vi "Update DUT Status.vi"(6 "Position":i32, 7 "Ignore State (true)":bool=TRUE, 8 "error in (no error)":errorcluster, 9 "BG Color":u32(colorbox), 10 "Message ('')":string, 11 "Application in":refnum<class "Application.lvclass">) -> (0 "error out":errorcluster, 3 "Application out":refnum<class "Application.lvclass">)   [LabVIEW 2017, in "Application.lvlib" / "Application.lvclass"]
doc: "Updates a specified position's status messge with the \"Message\" and \"BG Color\". If \"Ignore State\" is false it only updates the status if it's in the \"Ready\" or \"Testing\" state."
uses:
  Application.lvclass
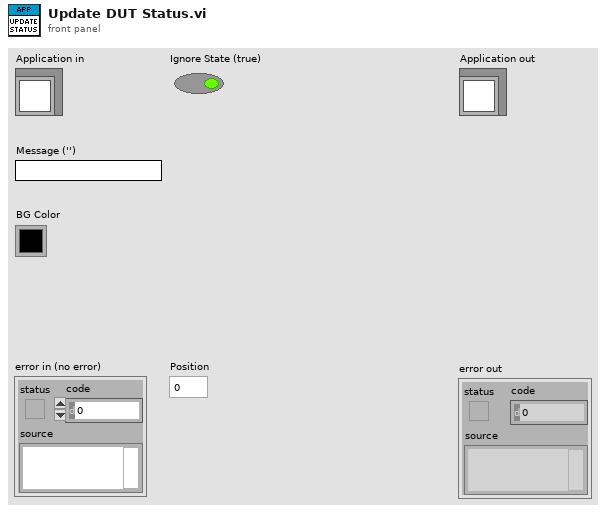
[diagram p1: front panel]
types:
  T1 = typedef "Application.lvlib/App Properties.lvclass/Class Properties -- Cluster.ctl" = cluster{"UUT Info":T2[], "Test Information":refnum<vi>, "Gold Board":refnum<class "Golden Board.lvclass">, "Test Recipe":refnum<class "Test Recipe.lvclass">, "Instruments":refnum<class "Instrument.lvclass">[], "Mode":T3, "Test Results":T4[], "Station Config":refnum<class "Station Config.lvclass">, "Variable Engine":refnum<class "Variable Engine.lvclass">}
  T2 = typedef "Application.lvlib/App Properties.lvclass/UUT Reference -- Cluster.ctl" = cluster{"Serial Number Reference":refnum<vi>, "Status Message Reference":refnum<vi>}
  T3 = typedef "Application.lvlib/Application.lvclass/Op Mode -- Enum.ctl" = u16
  T4 = typedef "Application.lvlib/App Properties.lvclass/Test Result -- Cluster.ctl" = cluster{"Position":i32, "Pass":bool, "Fail Codes":string}
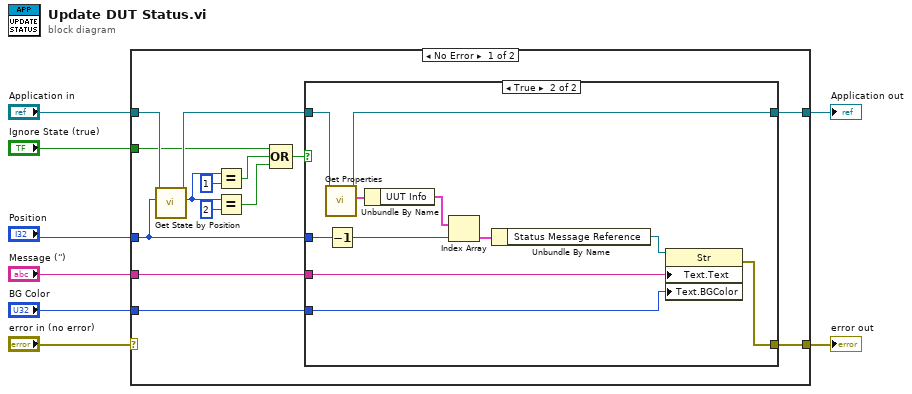
[diagram p0: block diagram]
diagram:
  n1 = case shown="No Error" "error in (no error)" {
    selector: "error in (no error)" -> [_ w36]
    tunnel: [w19 w36] -> w7
    tunnel: [w22 w35] -> w5
    tunnel: "Application in" -> [w18 w35]
    tunnel: "Message ('')" -> [w21 _]
    tunnel: "Position" -> [w9 _]
    tunnel: "BG Color" -> [w20 _]
    tunnel: "Ignore State (true)" -> [w13 _]
    frame No Error {
      n2 = call-dynamic "Get State by Position.vi"("Position"=w9, "Application in"=w18) -> ("State"=w14:u32, "Application out"=w17:refnum<class "Application.lvclass">)  [unwired: 7 in, 1 out]
      n3 = Equal?(x=w14, y=u32 1) -> (x = y?=w12:bool)
      n4 = Equal?(x=w14, y=u32 2) -> (x = y?=w11:bool)
      n5 = Compound Arithmetic op=OR(w13, w12, w11) -> (w10:bool)
      n6 = case shown="True" w10 {
        tunnel: [w23 w34] -> w22
        tunnel: w21 -> [_ w32]
        tunnel: w20 -> [_ w31]
        tunnel: [_ w30] -> w19
        tunnel: w17 -> [w23 w26]
        tunnel: w9 -> [_ w25]
        frame False {
        }
        frame True {
          n7 = call "Get Properties.vi"("Acrobat Template in"=w26) -> ("Class Properties"=w33:T1, "Acrobat Template out"=w34:refnum<class "Application.lvclass">)  [unwired: 8 in, 1 out]
          n8 = Decrement(x=w25) -> (x-1=w24:i32)
          n9 = Unbundle By Name(w33) -> ("UUT Info"=w29:T2[])
          n10 = Index Array(array=w29, index=w24) -> (element=w28:T2)
          n11 = Unbundle By Name(w28) -> ("Status Message Reference"=w27:refnum<vi>)
          n12 = property class="Str"(reference=w27, "Text.Text"=w32, "Text.BGColor"=w31) -> (error out=w30:errorcluster)  [unwired: 1 in, 1 out]
        }
      }
    }
    frame Error {
    }
  }
  "error out" <- w7
  "Application out" <- w5
